vi "Get XY Coordinates.vi"(8 "error in (no error)":errorcluster, 11 "VISA resource name":refnum<visa-resource-name>="GPIB1::11::INSTR") -> (0 "error out":errorcluster, 1 "X_Y":string, 2 "Y":string, 3 "X":string)   [LabVIEW 2013]
uses:
  Public/Documents/National Instruments/TestStand 2013/Components/Modules/NI_SemiconductorModule/Handlers/TEL_P-8_P-12XL/Source/TEL GPIB Command Set/TEL GPIB Command Set.lvlib
panel:
  out "return count":u32
  out "Prober XY":string
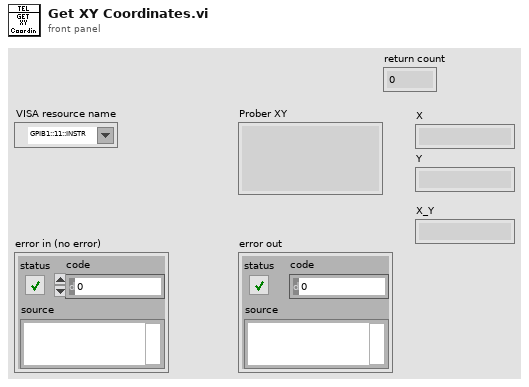
[diagram p1: front panel]
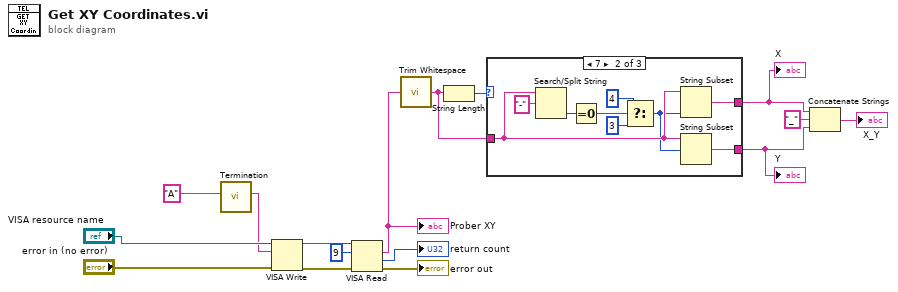
[diagram p0: block diagram]
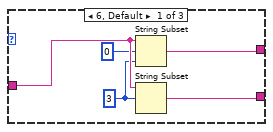
[diagram p2: hidden frame]
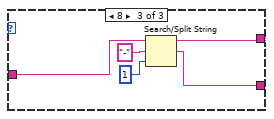
[diagram p3: hidden frame]
diagram:
  n1 = call "Termination.vi"("Input"="A" ("string")) -> ("Output"=w9:string)  [unwired: 10 in]
  n2 = VISA Write(VISA resource name="VISA resource name", write buffer=w9, error in (no error)="error in (no error)") -> (VISA resource name out=w14:refnum<visa-resource-name>, error out=w13:errorcluster)  [unwired: 1 out]
  n3 = VISA Read(VISA resource name=w14, byte count=u32 9, error in (no error)=w13) -> (read buffer=w6:string, return count=→"return count":u32, error out=→"error out":errorcluster)  [unwired: 1 out]
  "Prober XY" <- w6
  n4 = call <vilib>:"Trim Whitespace.vi"("string"=w6) -> ("trimmed string"=w7:string)  [unwired: 1 in]
  n5 = String Length(string=w7) -> (length=w8:i32)
  n6 = case shown="7" w8 {
    tunnel: w7 -> [w21 w24 w34]
    tunnel: [w19 w29 w32] -> w4
    tunnel: [w18 w22 w31] -> w3
    frame 6, Default {
      w17 = 3 ("length (rest)")
      n7 = String Subset(string=w21, offset (0)=0, length (rest)=w17) -> (substring=w19:string)
      n8 = String Subset(string=w21, offset (0)=w17) -> (substring=w18:string)  [unwired: 1 in]
    }
    frame 7 {
      n9 = Search/Split String(string=w24, search string/char (-)="-") -> (offset of match=w28:i32)  [unwired: 1 in, 2 out]
      n10 = Equal To 0?(x=w28) -> (x = 0?=w27:bool)
      n11 = Select(t=4 ("length (rest)"), s=w27, f=3 ("length (rest)")) -> (s? t:f=w23:i32)
      n12 = String Subset(string=w24, length (rest)=w23) -> (substring=w29:string)  [unwired: 1 in]
      n13 = String Subset(string=w24, offset (0)=w23) -> (substring=w22:string)  [unwired: 1 in]
    }
    frame 8 {
      n14 = Search/Split String(string=w34, search string/char (-)="-", offset (0)=1) -> (substring before match=w32:string, match + rest of string=w31:string)  [unwired: 1 out]
    }
  }
  "X" <- w4
  "Y" <- w3
  n15 = Concatenate Strings(w4, "_" ("string"), w3) -> (→"X_Y":string)
